vi "closeXML.vi"(8 "error in (no error)":errorcluster, 11 "NativeXML in":refnum<class "NativeXML.lvclass">) -> (0 "error out":errorcluster)   [LabVIEW 2011, in "Tools.lvlib" / "xml.lvlib" / "NativeXML.lvclass"]
uses:
  NativeXML.lvclass
  NativeXML.lvclass/NativeXML.ctl
  <vilib>/xml/Close Reference(Node).vi
  <vilib>/xml/NI_XML.lvlib
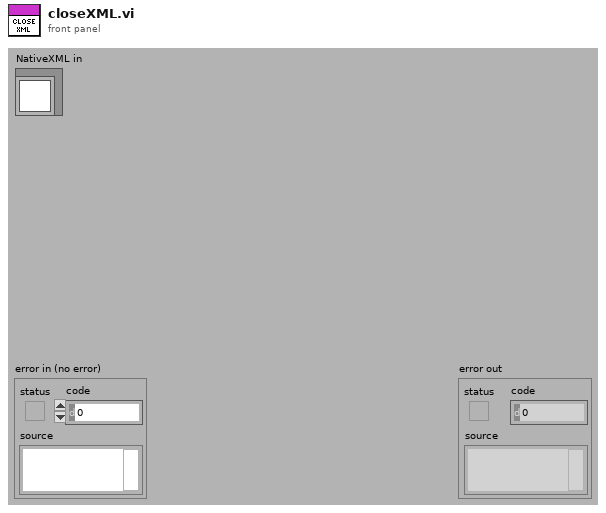
[diagram p1: front panel]
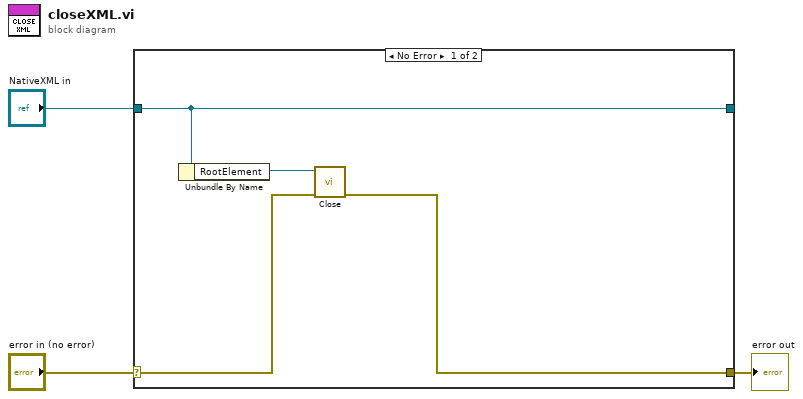
[diagram p0: block diagram]
diagram:
  n1 = case shown="No Error" "error in (no error)" {
    selector: "error in (no error)" -> [w5 w9]
    tunnel: [w4 w9] -> w2
    tunnel: [w7 w8] -> _
    tunnel: "NativeXML in" -> [w7 w8]
    frame No Error {
      n2 = Unbundle By Name(w7) -> ("RootElement"=w6:refnum<k20>)
      n3 = call-poly <vilib>:"Close.vi"("error in (no error)"=w5, "node"=w6) -> ("error out"=w4:errorcluster)  [unwired: 7 in]
    }
    frame Error {
    }
  }
  "error out" <- w2
